vi "ex_5.vi"() -> ()   [LabVIEW 2020]
uses:
  #typedef_FGV_LogsAction.ctl
  #typedef_Log.ctl
panel:
  out "Logs":string
  in  "Record Number":i32
  in  "Log":T1
  in  "Logs Action (GetList)":T2=enum."GetList"
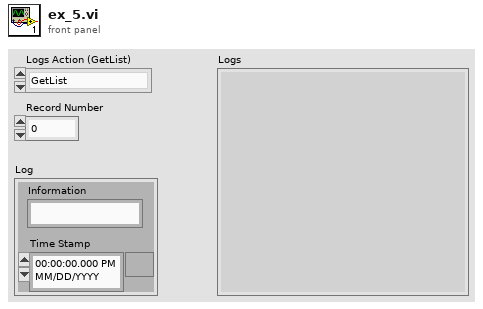
[diagram p1: front panel]
types:
  T1 = typedef "#typedef_Log.ctl" = cluster{"Information":string, "Time Stamp":timestamp}
  T2 = typedef "#typedef_FGV_LogsAction.ctl" = enum16{"ClearList", "AddRecord", "GetList"}
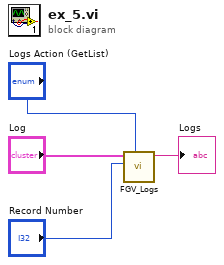
[diagram p0: block diagram]
diagram:
  n1 = call "FGV_Logs.vi"("Logs Action (GetList)"="Logs Action (GetList)", "Record Number"="Record Number", "Log"="Log") -> ("Logs"=→"Logs":string)  [unwired: 7 in, 1 out]
